vi "Write.vi"(5 "Username":string, 6 "Password":string, 7 "Address":string, 8 "Error In":errorcluster) -> (0 "Error Out":errorcluster)   [LabVIEW 2018, in "Tests.lvlib" / "SFTP File.lvlib"]
uses:
  SFTP File.lvlib
  src/Toolkit/API/SFTP File/API/Typedefs/Flags.ctl
  <vilib>/addons/_JKI Toolkits/Caraya/classes/Test/Test.lvclass
  <vilib>/addons/_JKI Toolkits/Caraya/classes/Assert/Assert.lvclass
  src/Toolkit/API/SFTP File/SFTP File.lvclass
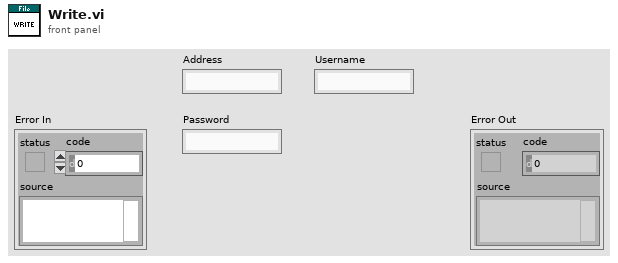
[diagram p1: front panel]
types:
  T1 = typedef "Toolkit.lvlib/SFTP File.lvclass/Flags.ctl" = cluster{"Read":bool, "Write":bool, "Append":bool, "Create":bool, "Truncate":bool, "Exclude":bool}
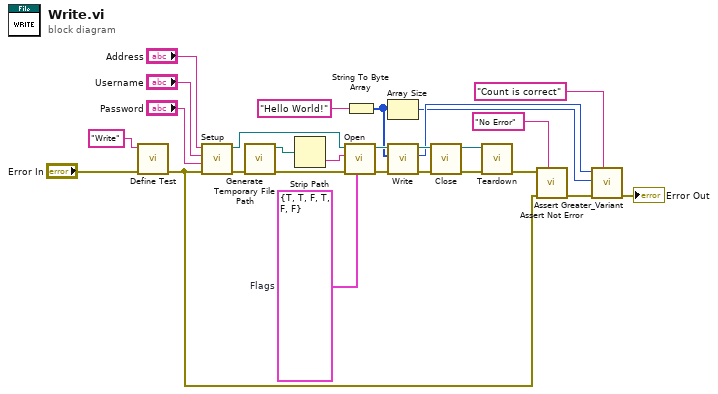
[diagram p0: block diagram]
diagram:
  w1 = T1 {"Read"=TRUE, "Write"=TRUE, "Append"=FALSE, "Create"=TRUE, "Truncate"=FALSE, "Exclude"=FALSE}  # Flags
  n1 = call <vilib>:"Define Test.vi"("error in (no error)"="Error In", "Label (VI Title)"="Write") -> ("error out"=w18:errorcluster)  [unwired: 9 in]
  n2 = call "Setup.vi"("Error In"=w18, "Password"="Password", "Username"="Username", "Address"="Address") -> ("Error Out"=w13:errorcluster, "SFTP"=w15:refnum<class "SFTP.lvclass">)  [unwired: 6 in]
  n3 = call <vilib>:"Generate Temporary File Path.vi"("error in (no error)"=w13) -> ("error out"=w12:errorcluster, "Unique Temporary File Path"=w11:path)  [unwired: 9 in]
  n4 = Strip Path(path=w11) -> (name=w10:string)  [unwired: 1 out]
  n5 = call "Open.vi"("Flags"=w1, "Error In"=w12, "Remote Path"=w10, "SFTP"=w15) -> ("Error Out"=w5:errorcluster, "SFTP File"=w9:refnum<class "SFTP File.lvclass">)  [unwired: 6 in]
  n6 = String To Byte Array(string="Hello World!") -> (unsigned byte array=w3:u8[])
  n7 = Array Size(array=w3) -> (size(s)=w2:i32)
  n8 = call "Write.vi"("Error In"=w5, "Data"=w3, "SFTP File In"=w9) -> ("Error Out"=w7:errorcluster, "Count"=w6:i64, "SFTP File Out"=w8:refnum<class "SFTP File.lvclass">)  [unwired: 6 in]
  n9 = call "Close.vi"("Error In"=w7, "SFTP File"=w8) -> ("Error Out"=w17:errorcluster, "SFTP"=w14:refnum<class "SFTP.lvclass">)  [unwired: 8 in]
  n10 = call "Teardown.vi"("Error In"=w17, "SFTP"=w14) -> ("Error Out"=w16:errorcluster)  [unwired: 9 in]
  n11 = call <vilib>:"Assert Not Error.vi"("Label"="No Error", "error in (no error)"=w18, "Not Error?"=w16) -> ("error out"=w24:errorcluster)  [unwired: 8 in]
  n12 = call <vilib>:"Assert Greater_Variant.vi"("Label"="Count is correct", "error in (no error)"=w24, "Y"=w2, "X"=w6) -> ("error out"=→"Error Out":errorcluster)  [unwired: 7 in]
